vi "sub_bonding-force.vi"(8 "error in":errorcluster caption="에러 입력(에러 없음)", 11 "sum of wf":waveform(dbl)) -> (0 "error out":errorcluster caption="에러 출력", 2 "Y max":dbl caption="Y 최대" format="%0.2f", 3 "high state level":dbl caption="높은 상태 레벨" format="%.2g")   [LabVIEW 2013]
uses:
  <vilib>/measure/mascope.llb/Amplitude and Levels 1 chan.vi
  <vilib>/measure/mamon.llb/Trigger Detection for 1 Channel.vi
  <vilib>/measure/NI_MAPro.lvlib
panel:
  out "웨이브폼 그래프":waveform(dbl)(graph)
  out "x-y":dbl
  out "Y min":dbl caption="Y 최소" format="%0.2f"
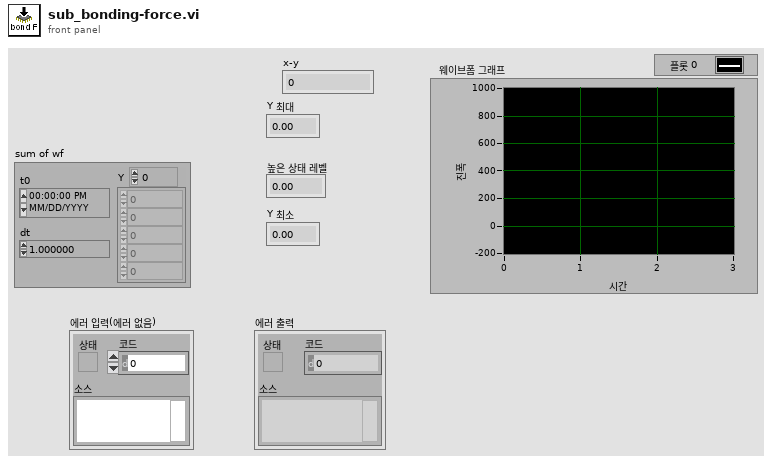
[diagram p1: front panel]
types:
  T1 = typedef "config_ctl.ctl" = cluster{"Trigger minlevel":dbl, "Lower Cut-Off":dbl, "Vacuum Trigger level":dbl, "state settings":cluster{"method":enum32{"histogram", "peak", "auto select"}, "histogram size":i32, "histogram method":enum16{"mode"}, "reserved":dbl}, "SPA-300 Setting":cluster{"Bonding force (g)":dbl, "Bonding time (ms)":dbl, "Pickup force (g)":dbl, "Pickup time (ms)":dbl, "Speed":enum16{"Slow", "Fast"}}}
  T2 = cluster{"method":enum32{"histogram", "peak", "auto select"}, "histogram size":i32, "histogram method":enum16{"mode"}, "reserved":dbl}
  T3 = typedef "UI_ctl.ctl" = cluster{"Heater temp":refnum<vi>, "Heater chart":refnum<vi>, "vacuum (kpa)":refnum<vi>, "Balance xy graph":refnum<vi>, "Strain chart w cal":refnum<vi>, "Pickup force":refnum<vi>, "Pickup time":refnum<vi>, "Force chart":refnum<vi>, "Trigger graph":refnum<vi>, "vacuum chart":refnum<vi>, "vacuum":refnum<vi>, "Strain raw graph":refnum<vi>, "Strain raw chart":refnum<vi>, "Bonding time":refnum<vi>, "Bonding force":refnum<vi>, "Balance":refnum<vi>, "Filtered force graph":refnum<vi>, "ROI intensity":refnum<vi>, "Heater_rt":refnum<vi>, "Tensile force":refnum<vi>, "Force rt":refnum<vi>}
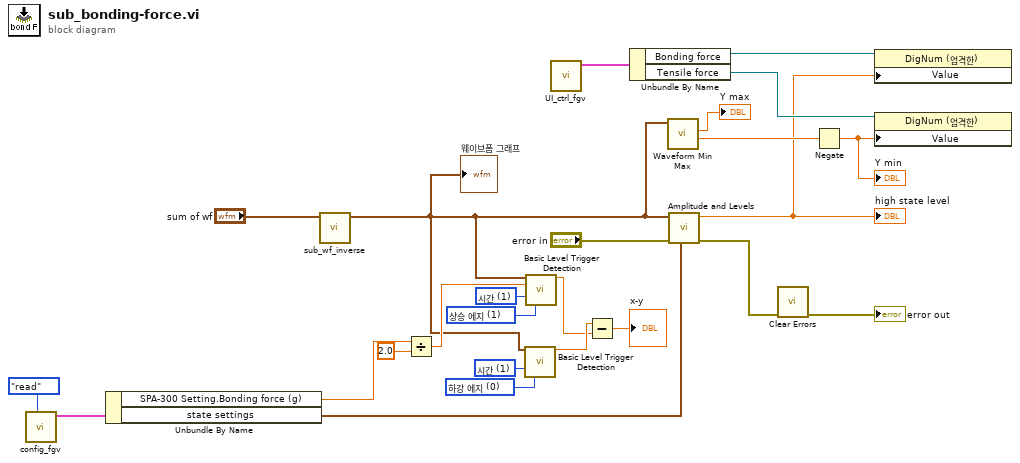
[diagram p0: block diagram]
diagram:
  w6 = u16 0 items=["하강 에지", "상승 에지"] ("trigger slope")
  w7 = u16 1 items=["인덱스", "시간"] ("location mode")
  w8 = u16 1 items=["하강 에지", "상승 에지"] ("trigger slope")
  w9 = u16 1 items=["인덱스", "시간"] ("location mode")
  n1 = call "config_fgv.vi"("cmd"=enum16{"write", "read", "ini"}."read") -> ("Config out"=w22:T1)  [unwired: 9 in, 1 out]
  n2 = Unbundle By Name(w22) -> ("SPA-300 Setting.Bonding force (g)"=w12:dbl, "state settings"=w23:T2)
  n3 = call "sub_wf_inverse.vi"("Trigger graph"="sum of wf") -> ("inverse graph"=w3:waveform(dbl))  [unwired: 10 in]
  "웨이브폼 그래프" <- w3
  n4 = Divide(x=w12, y=2.0) -> (x/y=w10:dbl)
  n5 = call-poly <vilib>:"Basic Level Trigger Detection.vi"("signal in"=w3, "location mode"=w7, "trigger slope"=w6) -> ("trigger location"=w2:dbl)  [unwired: 10 in, 2 out]
  n6 = call-poly <vilib>:"Basic Level Trigger Detection.vi"("signal in"=w3, "level"=w10, "location mode"=w9, "trigger slope"=w8) -> ("trigger location"=w1:dbl)  [unwired: 9 in, 2 out]
  n7 = call "UI_ctrl_fgv.vi"() -> ("UI cluster out"=w24:T3)  [unwired: 11 in]
  n8 = Subtract(x=w2, y=w1) -> (x-y=→"x-y":dbl)
  n9 = Unbundle By Name(w24) -> ("Bonding force"=w25:refnum<vi>, "Tensile force"=w17:refnum<vi>)
  n10 = call <vilib>:"Waveform Min Max.vi"("waveform in"=w3) -> ("Y min"=w16:dbl, "Y max"=→"Y max":dbl)  [unwired: 5 in, 4 out]
  n11 = call-poly <vilib>:"Amplitude and Levels.vi"("state settings"=w23, "error in (no error)"="error in", "signal in"=w3) -> ("error out"=w19:errorcluster, "amplitude"=w14:dbl)  [unwired: 5 in, 2 out]
  "high state level" <- w14
  n12 = call <vilib>:"Clear Errors.vi"("error in (no error)"=w19) -> ("error out"=→"error out":errorcluster)  [unwired: 6 in]
  n13 = Negate(x=w16) -> (-x=w15:dbl)
  "Y min" <- w15
  n14 = property class="DigNum (엄격한)"(reference=w25, "Value"=w14) -> ()  [unwired: 1 in, 2 out]
  n15 = property class="DigNum (엄격한)"(reference=w17, "Value"=w15) -> ()  [unwired: 1 in, 2 out]
